vi "sub_ECC_infocom.vi"() -> ()   [LabVIEW 2021]
uses:
  system stop.vi
  <vilib>/gmath/NI_Gmath.lvlib
panel:
  out "correlation coefficient r":dbl format="%.7g"
  out "Size":dbl
  out "Filtered Signal":dbl[](array[numeric])
  out "output array size":u32
  out "SDR1 Key":u8[](array[numeric])
  out "SDR2 Key":u8[](array[numeric])
  out "CR rate":dbl[](array[numeric])
  in  "Quantization rate":dbl
  in  "Python path":path=path "C:/Users/prashanth/Documents/GitHub/CR_Quantization/labview_demo_continuous.py"
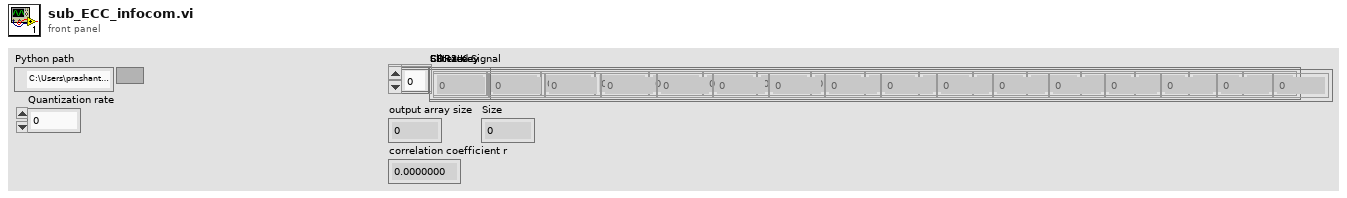
[diagram p1: front panel]
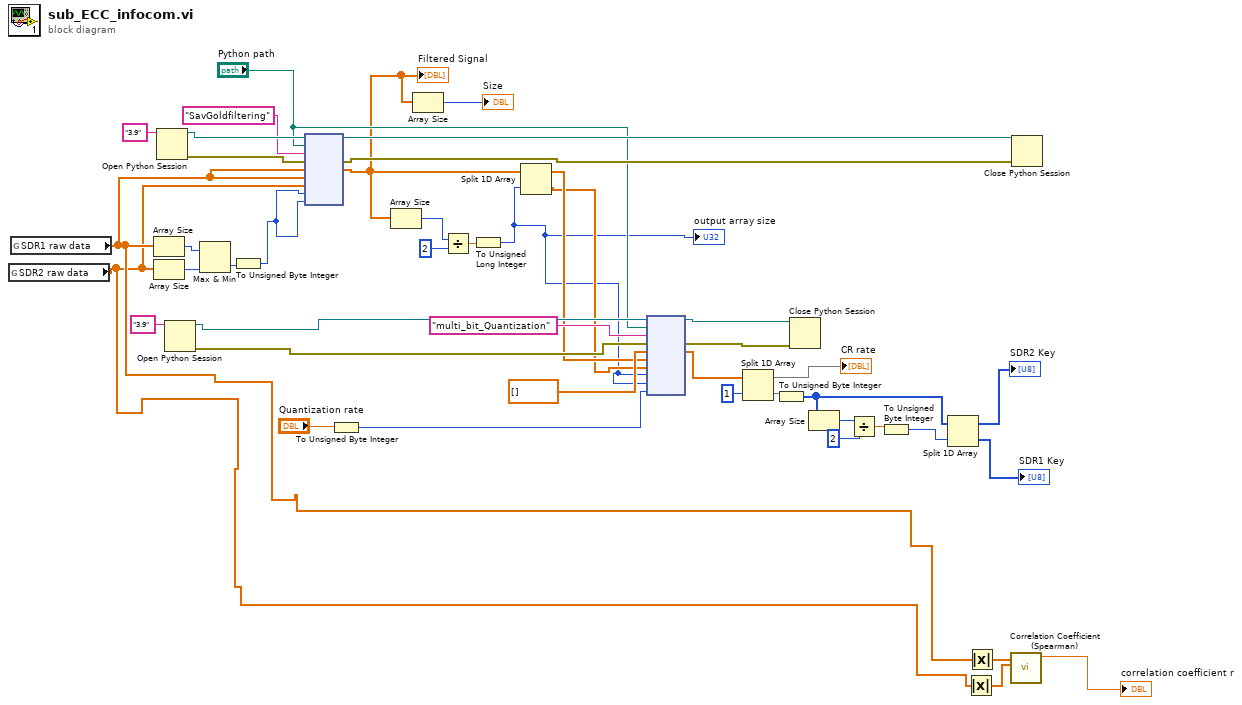
[diagram p0: block diagram]
diagram:
  n1 = global read "system stop.vi" "SDR2 raw data"() -> (w4:dbl[])
  n2 = global read "system stop.vi" "SDR1 raw data"() -> (w5:dbl[])
  n3 = Array Size(array=w5) -> (size(s)=w19:i32)
  n4 = Array Size(array=w4) -> (size(s)=w20:i32)
  n5 = Open Python Session(python version="3.9" ("Python version")) -> (session out=w44:refnum<k35>, error out=w42:errorcluster)  [unwired: 2 in]
  n6 = Open Python Session(python version="3.9" ("Python version")) -> (session out=w35:refnum<k35>, error out=w34:errorcluster)  [unwired: 2 in]
  n7 = Max & Min(x=w19, y=w20) -> (min(x,y)=w12:i32)  [unwired: 1 out]
  n8 = To Unsigned Byte Integer(number=w12) -> (unsigned 8bit integer=w11:u8)
  n9 = node(w44, "Python path", "SavGoldfiltering" ("function name"), w42, w5, w5, w4, w11, w11) -> (w43:refnum<k35>, w29:errorcluster, w14:dbl[])  [unwired: 4 in, 2 out]
  "Filtered Signal" <- w14
  n10 = To Unsigned Byte Integer(number="Quantization rate") -> (unsigned 8bit integer=w9:u8)
  n11 = Array Size(array=w14) -> (size(s)=w30:i32)
  n12 = Array Size(array=w14) -> (size(s)=→"Size":i32)
  n13 = Divide(x=w30, y=2) -> (x/y=w38:dbl)
  n14 = To Unsigned Long Integer(number=w38) -> (unsigned 32bit integer=w17:u32)
  "output array size" <- w17
  n15 = Split 1D Array(array=w14, index=w17) -> (first subarray=w32:dbl[], second subarray=w31:dbl[])
  n16 = node(w35, "Python path", "multi_bit_Quantization" ("function name"), w34, dbl[] [], w32, w31, w17, w17, w9) -> (w28:refnum<k35>, w27:errorcluster, w25:dbl[])  [unwired: 5 in, 2 out]
  n17 = Split 1D Array(array=w25, index=1) -> (first subarray=→"CR rate":dbl[], second subarray=w7:dbl[])
  n18 = To Unsigned Byte Integer(number=w7) -> (unsigned 8bit integer=w6:u8[])
  n19 = Close Python Session(session in=w28, error in=w27) -> ()  [unwired: 1 out]
  n20 = Array Size(array=w6) -> (size(s)=w24:i32)
  n21 = Divide(x=w24, y=2) -> (x/y=w16:dbl)
  n22 = To Unsigned Byte Integer(number=w16) -> (unsigned 8bit integer=w15:u8)
  n23 = Split 1D Array(array=w6, index=w15) -> (first subarray=→"SDR2 Key":u8[], second subarray=→"SDR1 Key":u8[])
  n24 = Absolute Value(x=w4) -> (abs(x)=w2:dbl[])
  n25 = Absolute Value(x=w5) -> (abs(x)=w3:dbl[])
  n26 = call <vilib>:"Correlation Coefficient (Spearman).vi"("Y"=w2, "X"=w3) -> ("correlation coefficient r"=→"correlation coefficient r":dbl)  [unwired: 8 in, 1 out]
  n27 = Close Python Session(session in=w43, error in=w29) -> ()  [unwired: 1 out]
